vi "CB Flywheel Model.vi"(4 "k":dbl=1.0, 5 "J (moment of intertia kgm^2)":dbl, 6 "encoder?":bool=TRUE, 7 "G (gear ratio)":dbl, 8 "dt":dbl=-1.0, 10 "num motors":i32=1, 11 "Motor ID":T3) -> (3 "State Space Model":T1)   [LabVIEW 2020]
uses:
  Motors/CB Motor ID.ctl
  CB State Space.ctl
  <vilib>/Analysis/Matrix/Datatypes/RealMatrix.ctl
  <vilib>/Analysis/Matrix/NI_Matrix.lvlib
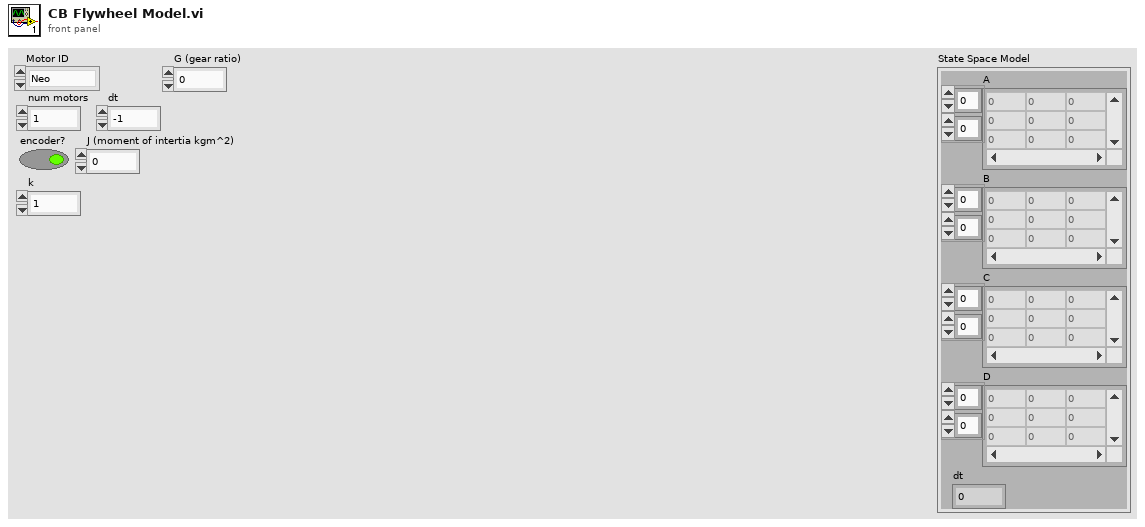
[diagram p1: front panel]
types:
  T1 = typedef "CB State Space.ctl" = cluster{"A":T2, "B":T2, "C":T2, "D":T2, "dt":dbl}
  T2 = typedef "NI_Matrix.lvlib/RealMatrix.ctl" = dbl[][]
  T3 = typedef "CB Motor ID.ctl" = enum16{"Neo", "Neo 550", "Falcon 500", "775pro"}
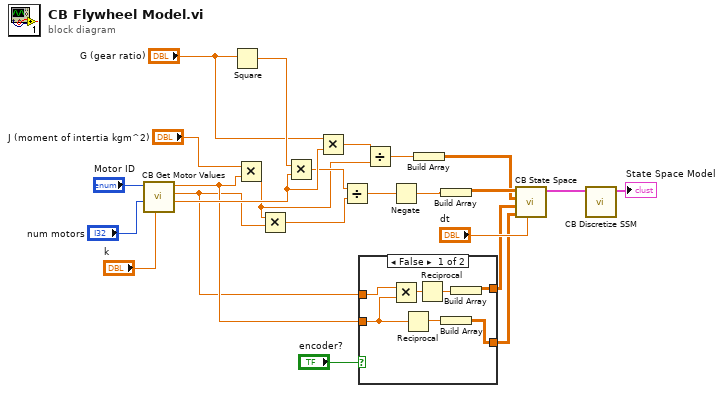
[diagram p0: block diagram]
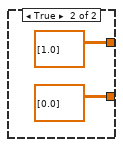
[diagram p2: hidden frame]
diagram:
  n1 = call "CB Get Motor Values.vi"("k"="k", "num motors"="num motors", "Motor ID"="Motor ID") -> ("Kt"=w17:dbl, "Kv"=w7:dbl, "R"=w8:dbl)  [unwired: 5 in, 1 out]
  n2 = Square(x="G (gear ratio)") -> (x^2=w18:dbl)
  n3 = Multiply(x="J (moment of intertia kgm^2)", y=w8) -> (x*y=w11:dbl)
  n4 = Multiply(x=w11, y=w7) -> (x*y=w13:dbl)
  n5 = Multiply(x=w18, y=w17) -> (x*y=w14:dbl)
  n6 = Multiply(x="G (gear ratio)", y=w17) -> (x*y=w12:dbl)
  n7 = Divide(x=w14, y=w13) -> (x/y=w5:dbl)
  n8 = case shown="False" "encoder?" {
    tunnel: [w25 T2 [[1.0]] ("C")] -> w21
    tunnel: [w30 T2 [[0.0]] ("D")] -> w20
    tunnel: w8 -> [w29 _]
    tunnel: w7 -> [w28 _]
    frame False {
      n9 = Multiply(x=w28, y=w29) -> (x*y=w27:dbl)
      n10 = Reciprocal(x=w29) -> (1/x=w31:dbl)
      n11 = Reciprocal(x=w27) -> (1/x=w26:dbl)
      n12 = Build Array(w31) -> (w30:T2)
      n13 = Build Array(w26) -> (w25:T2)
    }
    frame True {
    }
  }
  n14 = Divide(x=w12, y=w11) -> (x/y=w6:dbl)
  n15 = Negate(x=w5) -> (-x=w4:dbl)
  n16 = Build Array(w6) -> (w9:T2)
  n17 = Build Array(w4) -> (w10:T2)
  n18 = call "CB State Space.vi"("dt"="dt", "D"=w20, "C"=w21, "B"=w9, "A"=w10) -> ("State Space Model"=w3:T1)  [unwired: 5 in, 1 out]
  n19 = call "CB Discretize SSM.vi"("Cont SSM"=w3) -> ("State Space Model"=→"State Space Model":T1)  [unwired: 10 in]
